vi "DefineGrid.vi"(8 "error in":T2, 11 "Cluster":T1 {"YCoordinates" format="%#_g µm"; "XCoordinates" format="%#_g µm"}) -> (0 "error out":T2, 3 "Output Cluster":T1 {"YCoordinates" format="%#_g µm"; "XCoordinates" format="%#_g µm"})   [LabVIEW 2016]
doc: "This VI creates a grid which is then processed point by point in path mode when started with StartPathmode.vi. The input parameters are:\n- NumberOfPointsX (integer) [without restraint]\n- NumberOfPointsY (integer) [without restraint]\n- CoordX [µm] (Array of floats) [without restraint]\n- CoordY [µm] (Array of floats) [without restraint]\nThe grid is defined by three points, which are passed by the arrays CoordX and CoordY. The first point should be passed at index 0 in the arrays CoordX and CoordY defining the origin point of the grid. The second point passed at index 1 defines the furthest away point from the origin point on the x-axis. The third point passed at index 2 defines the furthest away point on the y-axis.\nBy passing -Inf (float) or -2147483648 (integer) the corresponding value will be read out."
uses:
  Controls/Grid_Parameters.ctl
  Controls/Error_Out.ctl
  Files_ASC500/DLL/ASC500_RemoteControlV27.dll
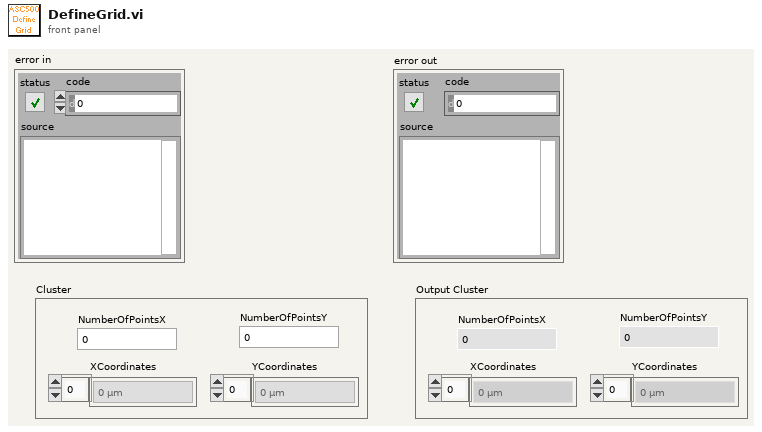
[diagram p1: front panel]
types:
  T1 = typedef "Grid_Parameters.ctl" = cluster{"NumberOfPointsX":i32, "NumberOfPointsY":i32, "XCoordinates":sgl[], "YCoordinates":sgl[]}
  T2 = typedef "Error_Out.ctl" = errorcluster
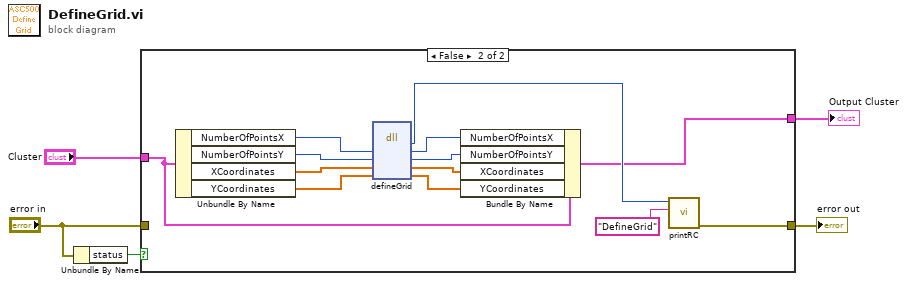
[diagram p0: block diagram]
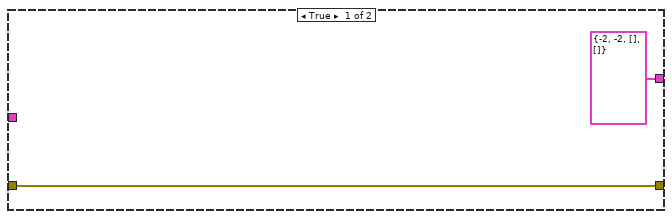
[diagram p2: hidden frame]
diagram:
  n1 = Unbundle By Name("error in") -> ("status"=w5:bool)
  n2 = case shown="False" w5 {
    tunnel: "Cluster" -> [_ w13]
    tunnel: "error in" -> [w7 _]
    tunnel: [w7 w20] -> w2
    tunnel: [T1 {"NumberOfPointsX"=-2, "NumberOfPointsY"=-2, "XCoordinates"=[], "YCoordinates"=[]} ("Cluster") w8] -> w1
    frame True {
    }
    frame False {
      n3 = Unbundle By Name(w13) -> ("NumberOfPointsX"=w17:i32, "NumberOfPointsY"=w16:i32, "XCoordinates"=w15:sgl[], "YCoordinates"=w14:sgl[])
      n4 = dll-call lib="G:/SCMOperations/Share/ELE/Produkt Information/ASC500/04 Remote Control/02 development versions/2018Nov06/Files_ASC500/DLL/ASC500_RemoteControlV27.dll" fn="defineGrid"("numberOfPointsX"=w17, "NumberOfPointsY"=w16, "CoordX"=w15, "CoordY"=w14) -> ("return type"=w19:i32, "numberOfPointsX"=w9:i32, "NumberOfPointsY"=w12:i32, "CoordX"=w11:sgl[], "CoordY"=w10:sgl[])  [unwired: 3 in, 2 out]
      n5 = Bundle By Name(cluster=w13, "NumberOfPointsX"=w9, "NumberOfPointsY"=w12, "XCoordinates"=w11, "YCoordinates"=w10) -> (w8:T1)
      n6 = call "printRC.vi"("additional information"="DefineGrid", "RC"=w19) -> ("error out"=w20:T2)  [unwired: 9 in]
    }
  }
  "error out" <- w2
  "Output Cluster" <- w1
